vi "Loop.vi"(8 "error in (no error)":errorcluster, 11 "FHPP in":refnum<class "FHPP.lvclass">) -> (0 "error out":errorcluster, 3 "FHPP out":refnum<class "FHPP.lvclass">)   [LabVIEW 2022 SP3, in "FHPP.lvclass"]
uses:
  FHPP.lvclass
  FHPP.lvclass/FHPP.ctl
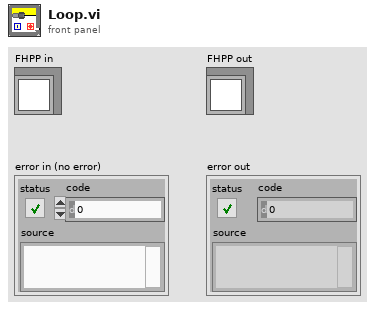
[diagram p1: front panel]
types:
  T1 = typedef "FHPP.lvclass/Operating Mode.ctl" = enum16{"Record Selection", "Direct Mode", "Reserved 1", "Reserved 2"}
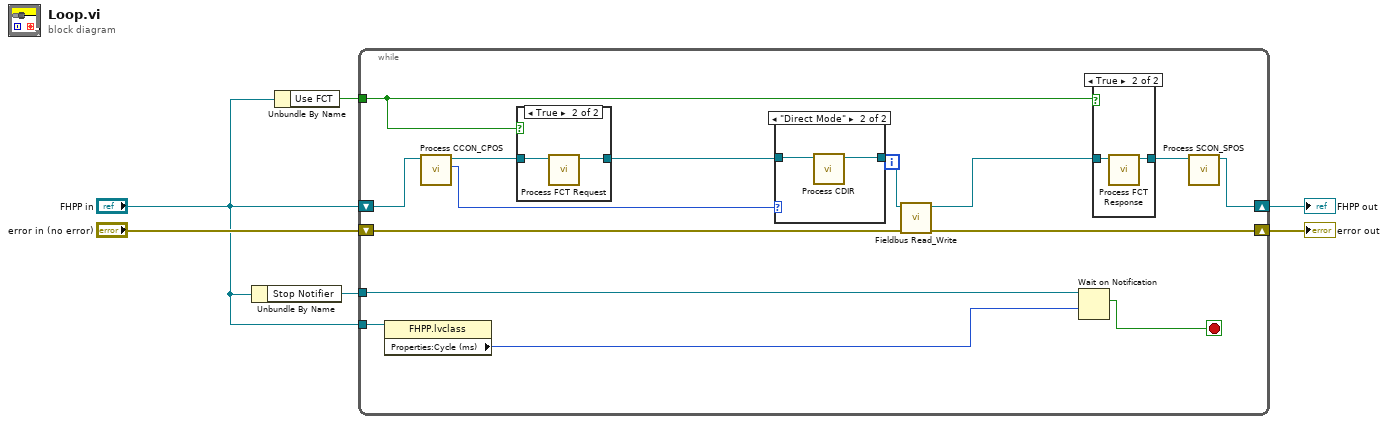
[diagram p0: block diagram]
diagram:
  n1 = Unbundle By Name("FHPP in") -> ("Stop Notifier"=w6:refnum<notifier>)
  n2 = Unbundle By Name("FHPP in") -> ("Use FCT"=w5:bool)
  n3 = while {
    tunnel: w5 -> [w14]
    shift-right: [w17] -> w3
    shift-left: "error in (no error)" -> [w18]
    shift-right: [w16] -> w4
    shift-left: "FHPP in" -> [w15]
    tunnel: w6 -> [w13]
    tunnel: "FHPP in" -> [w11]
    stop <- w12 stop-if-true
    n4 = property class="FHPP.lvclass"(reference=w11) -> ("Properties:Cycle (ms)"=w10:i32)  [unwired: 1 in, 2 out]
    n5 = call "Process CCON_CPOS.vi"("FHPP in"=w15) -> ("Desired Operating Mode"=w7:T1, "FHPP out"=w21:refnum<class "FHPP.lvclass">)  [unwired: 9 in]
    n6 = case shown="True" w14 {
      tunnel: w21 -> [w28 w30]
      tunnel: [w28 w29] -> w8
      frame False {
      }
      frame True {
        n7 = call "Process FCT Request.vi"("FHPP in"=w30) -> ("FHPP out"=w29:refnum<class "FHPP.lvclass">)  [unwired: 10 in]
      }
    }
    n8 = case shown="\"Direct Mode\"" w7 {
      tunnel: [w22 w23] -> w9
      tunnel: w8 -> [w22 w24]
      frame Default {
      }
      frame "Direct Mode" {
        n9 = call "Process CDIR.vi"("FHPP in"=w24) -> ("FHPP out"=w23:refnum<class "FHPP.lvclass">)  [unwired: 10 in]
      }
    }
    n10 = call "Fieldbus Read_Write.vi"("error in (no error)"=w18, "FHPP in"=w9) -> ("error out"=w17:errorcluster, "FHPP out"=w20:refnum<class "FHPP.lvclass">)  [unwired: 8 in]
    n11 = Wait on Notification(notifier=w13, timeout in ms (-1)=w10) -> (notification=w12:bool)  [unwired: 2 in, 3 out]
    n12 = case shown="True" w14 {
      tunnel: w20 -> [w25 w27]
      tunnel: [w25 w26] -> w19
      frame False {
      }
      frame True {
        n13 = call "Process FCT Response.vi"("FHPP in"=w27) -> ("FHPP out"=w26:refnum<class "FHPP.lvclass">)  [unwired: 10 in]
      }
    }
    n14 = call "Process SCON_SPOS.vi"("FHPP in"=w19) -> ("FHPP out"=w16:refnum<class "FHPP.lvclass">)  [unwired: 10 in]
  }
  "FHPP out" <- w4
  "error out" <- w3
